vi "Handle New Data.vi"(8 "error in (no error)":errorcluster, 10 "New Data":T1, 11 "Data Processor Module in":refnum<class "Data Processor Module.lvclass">) -> (0 "error out":errorcluster, 3 "Data Processor Module out":refnum<class "Data Processor Module.lvclass">)   [LabVIEW 2020, in "VolatusData.lvlib" / "Data Processor Module.lvclass"]
uses:
  Data Processor Module.lvclass
  C:/dev/lv20CE/relink/lv-volatus/Volatus/Module/Module.lvclass
  New Data.ctl
  Data Processor Module.lvclass/Data Processor Module.ctl
  Scaling/Scaling.lvclass/Scaling.ctl
  Volatus/MessageQ/MessageQ.lvclass/MessageQ.ctl
  Volatus/Module/Module.lvclass/Module.ctl
  Volatus/VolatusAPI/VolatusAPI.lvclass/VolatusAPI.ctl
  Scaling/Scale Channel Data.vi
  Volatus/MessageQ/Send.vi
  <vilib>/Analysis/baseanly.llb/Mean.vi
  <vilib>/Analysis/baseanly.llb/Mean (DBL).vi
  <vilib>/Utility/High Resolution Relative Seconds.vi
  Volatus/Module/Publish Group.vi
  Scaling/Scale Channel (Array).vi
  Volatus/VolatusAPI/Publish Group.vi
  Scaling/Polynomial Remove Trailing Zeros.vi
  Scaling/Expo Scale Array.vi
  lv-vecto/Vecto/Group DBL/Group DBL.lvclass
  C:/dev/lv20CE/relink/lv-vecto/Vecto/Group/Group.lvclass
  lv-vecto/Vecto/Group DBL/Update Values.vi
  lv-vecto/Vecto/RemoteDataService/Publish Group.vi
  VolatusData.lvlib
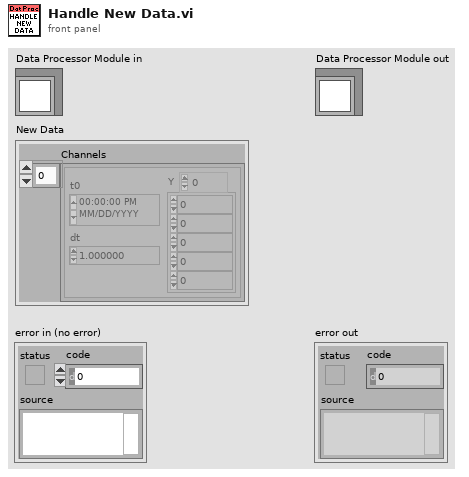
[diagram p1: front panel]
types:
  T1 = typedef "VolatusData.lvlib/New Data.ctl" = cluster{"Channels":waveform(dbl)[]}
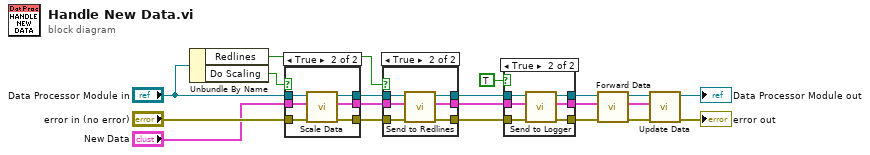
[diagram p0: block diagram]
diagram:
  n1 = Unbundle By Name("Data Processor Module in") -> ("Redlines"=w16:bool, "Do Scaling"=w19:bool)
  n2 = case shown="True" w19 {
    tunnel: "Data Processor Module in" -> [w23 w29]
    tunnel: [w23 w28] -> w18
    tunnel: "New Data" -> [w22 w27]
    tunnel: [w22 w26] -> w17
    tunnel: "error in (no error)" -> [w21 w25]
    tunnel: [w21 w24] -> w10
    frame False {
    }
    frame True {
      n3 = call "Scale Data.vi"("error in (no error)"=w25, "Data"=w27, "Data Processor Module in"=w29) -> ("error out"=w24:errorcluster, "Scaled Data"=w26:T1, "Data Processor Module out"=w28:refnum<class "Data Processor Module.lvclass">)  [unwired: 6 in]
    }
  }
  n4 = case shown="True" w16 {
    tunnel: w18 -> [w32 w38]
    tunnel: [w32 w37] -> w15
    tunnel: w17 -> [w31 w36]
    tunnel: [w31 w33] -> w14
    tunnel: w10 -> [w30 w35]
    tunnel: [w30 w34] -> w9
    frame False {
    }
    frame True {
      n5 = call "Send to Redlines.vi"("error in (no error)"=w35, "Data"=w36, "Data Processor Module in"=w38) -> ("error out"=w34:errorcluster, "Data dup"=w33:T1, "Data Processor Module out"=w37:refnum<class "Data Processor Module.lvclass">)  [unwired: 6 in]
    }
  }
  n6 = case shown="True" TRUE {
    tunnel: w15 -> [w41 w47]
    tunnel: w14 -> [w40 w46]
    tunnel: [w41 w45] -> w4
    tunnel: [w40 w44] -> w2
    tunnel: w9 -> [w39 w43]
    tunnel: [w39 w42] -> w8
    frame False {
    }
    frame True {
      n7 = call "Send to Logger.vi"("error in (no error)"=w43, "Data"=w46, "Data Processor Module in"=w47) -> ("error out"=w42:errorcluster, "Data dup"=w44:T1, "Data Processor Module out"=w45:refnum<class "Data Processor Module.lvclass">)  [unwired: 6 in]
    }
  }
  n8 = call "Forward Data.vi"("error in (no error)"=w8, "Data"=w2, "Data Processor Module in"=w4) -> ("error out"=w5:errorcluster, "Data dup"=w1:T1, "Data Processor Module out"=w3:refnum<class "Data Processor Module.lvclass">)  [unwired: 6 in]
  n9 = call "Update Data.vi"("error in (no error)"=w5, "Data"=w1, "Data Processor Module in"=w3) -> ("error out"=→"error out":errorcluster, "Data Processor Module out"=→"Data Processor Module out":refnum<class "Data Processor Module.lvclass">)  [unwired: 7 in]
